vi "Initialize with Switch Parameters Core.vi"(8 "error in (no error)":errorcluster, 10 "Switch Parameters in":refnum<class "Abstract Switch Init Parameters.lvclass">, 11 "SLSC Switch Consumer in":refnum<class "SLSC Switch Consumer.lvclass">) -> (0 "error out":errorcluster, 3 "SLSC Switch Consumer out":refnum<class "SLSC Switch Consumer.lvclass">)   [LabVIEW 2017, in "SLSC Switch Messaging.lvlib" / "SLSC Switch Consumer.lvclass"]
uses:
  SLSC Switch Consumer.lvclass
  SLSC-Switch-Simulator/Includes/CDMessaging.lvlibp/Switch/Abstract Switch Init Parameters/Abstract Switch Init Parameters.lvclass
  SLSC Switch Init Parameters/SLSC Switch Init Parameters.lvclass
  C:/dev/CustomDevice/SLSC-Switch-Simulator/Includes/CDMessaging.lvlibp/Switch/Abstract Switch Init Parameters/Abstract Switch Init Parameters.lvclass
  SLSC Switch Consumer.lvclass/SLSC Switch Consumer.ctl
  <vilib>/SLSC_Switch/Initialize with Topology (Device).vi
  Simulated Connection Monitor.vi
  <vilib>/SLSC_Switch/Initialize with Topology (Simulate).vi
  <vilib>/SLSC_Switch/SLSC Switch.lvlib
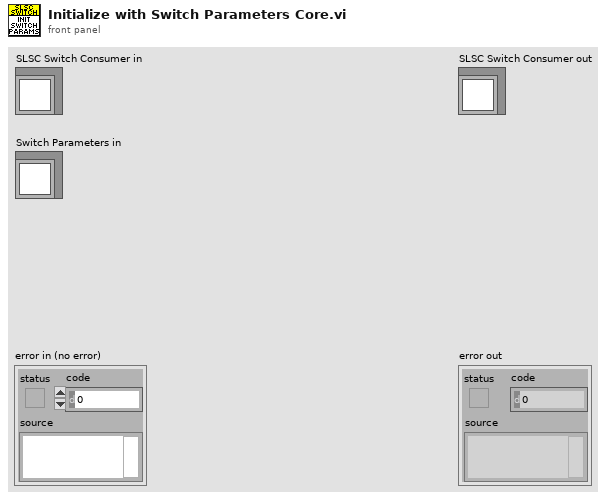
[diagram p1: front panel]
types:
  T1 = typedef "nislscslSession.ctl" = refnum<k20>
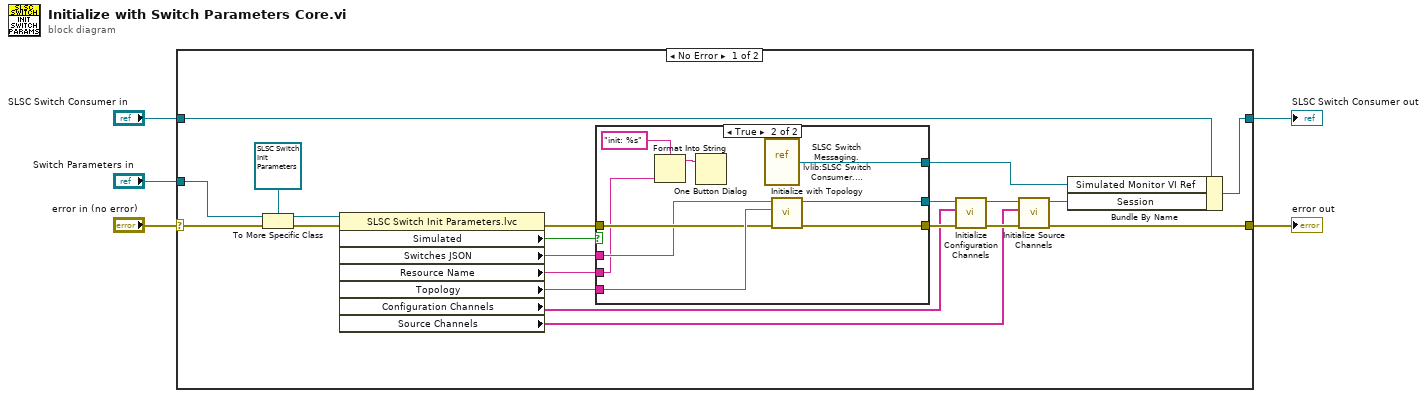
[diagram p0: block diagram]
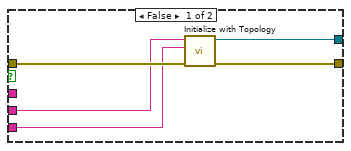
[diagram p2: hidden frame]
diagram:
  n1 = case shown="No Error" "error in (no error)" {
    selector: "error in (no error)" -> [w18 w42]
    tunnel: [w11 w42] -> w4
    tunnel: [w26 w41] -> w1
    tunnel: "SLSC Switch Consumer in" -> [w8 w41]
    tunnel: "Switch Parameters in" -> [w21 _]
    frame No Error {
      n2 = To More Specific Class(target class=refnum<class "SLSC Switch Init Parameters.lvclass"> refnum ("SLSC Switch Messaging.lvlib:SLSC Switch Init Parameters.lvclass"), reference=w21, error in=w18) -> (specific class reference=w19:refnum<class "SLSC Switch Init Parameters.lvclass">, error out=w17:errorcluster)
      n3 = property class="SLSC Switch Init Parameters.lvc"(reference=w19, error in=w17) -> (error out=w24:errorcluster, "Simulated"=w23:bool, "Switches JSON"=w25:string, "Resource Name"=w6:string, "Topology"=w22:string, "Configuration Channels"=w9:string[], "Source Channels"=w10:string[])  [unwired: 1 out]
      n4 = case shown="True" w23 {
        tunnel: w25 -> [_ w34]
        tunnel: [w31 w40] -> w13
        tunnel: [w30 w39] -> w16
        tunnel: w24 -> [w29 w37]
        tunnel: w6 -> [w28 w32]
        tunnel: w22 -> [w27 w38]
        tunnel: [_ w36] -> w7
        frame False {
          n5 = call-poly <vilib>:"Initialize with Topology.vi"("error in (no error)"=w29, "topology"=w27, "device"=w28) -> ("error out"=w31:errorcluster, "session out"=w30:T1)  [unwired: 7 in]
        }
        frame True {
          n6 = Format Into String(format string="init: %s", w32) -> (resulting string=w33:string)  [unwired: 2 in, 1 out]
          n7 = One Button Dialog(message=w33) -> ()  [unwired: 1 in, 1 out]
          n8 = vi-ref "SLSC Switch Messaging.lvlib:SLSC Switch Consumer.lvclass:Simulated Connection Monitor.vi"() -> (w36:refnum<vi>)
          n9 = call-poly <vilib>:"Initialize with Topology.vi"("error in (no error)"=w37, "topology"=w38, "switches json"=w34) -> ("error out"=w40:errorcluster, "session out"=w39:T1)  [unwired: 7 in]
        }
      }
      n10 = call "Initialize Configuration Channels.vi"("error in (no error)"=w13, "Configuration Channels"=w9, "Session in"=w16) -> ("error out"=w12:errorcluster, "Session out"=w15:T1)  [unwired: 7 in]
      n11 = call "Initialize Source Channels.vi"("error in (no error)"=w12, "Source Channels"=w10, "Session in"=w15) -> ("error out"=w11:errorcluster, "Session out"=w14:T1)  [unwired: 7 in]
      n12 = Bundle By Name(cluster=w8, "Simulated Monitor VI Ref"=w7, "Session"=w14) -> (w26:refnum<class "SLSC Switch Consumer.lvclass">)
    }
    frame Error {
    }
  }
  "error out" <- w4
  "SLSC Switch Consumer out" <- w1
